vi "Upd Full Scale Range.vi"(8 "error in (no error)":errorcluster, 10 "Full Scale Range":dbl, 11 "FC2901 in":refnum<class "FC2901.lvclass">) -> (0 "error out":errorcluster, 3 "FC2901 out":refnum<class "FC2901.lvclass">)   [LabVIEW 2021, in "FC2901.lvclass"]
uses:
  FC2901.lvclass
  FC2901.lvclass/FC2901.ctl
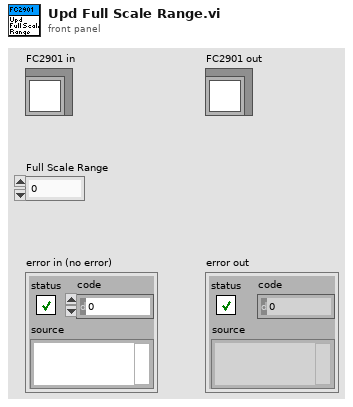
[diagram p1: front panel]
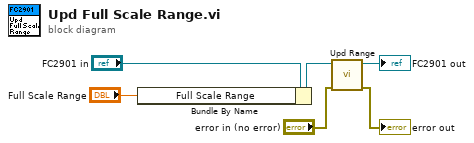
[diagram p0: block diagram]
diagram:
  n1 = Bundle By Name(cluster="FC2901 in", "Full Scale Range"="Full Scale Range") -> (w3:refnum<class "FC2901.lvclass">)
  n2 = call "Upd Range.vi"("error in (no error)"="error in (no error)", "C100L in"=w3) -> ("error out"=→"error out":errorcluster, "C100L out"=→"FC2901 out":refnum<class "FC2901.lvclass">)  [unwired: 8 in]
